vi "Remove All Aliases.vi"(8 "error in (no error)":errorcluster, 11 "Aliases Ref in":T1 format="%.0x") -> (0 "error out":errorcluster, 1 "Removed":bool, 3 "Aliases Ref out":T1 format="%.0x")   [LabVIEW 2017, in "Switch Scripting.lvlib"]
uses:
  Switch Scripting.lvlib
  <vilib>/NI Veristand/Custom Device API/Custom Device Item Ref.ctl
  <vilib>/NI VeriStand/Custom Device API/Custom Device API.lvlib
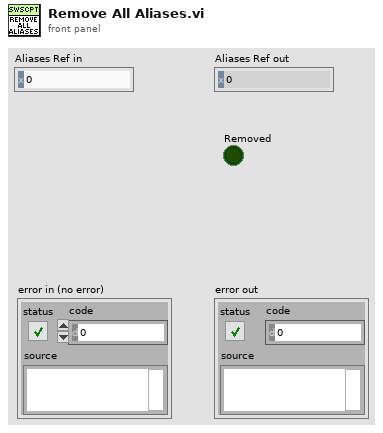
[diagram p1: front panel]
types:
  T1 = typedef "Custom Device API.lvlib/Custom Device Item Ref.ctl" = u64
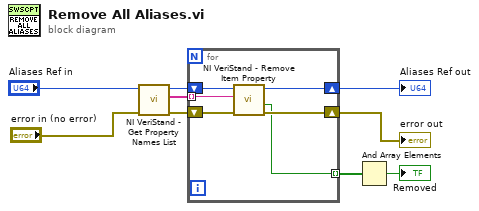
[diagram p0: block diagram]
diagram:
  n1 = call <vilib>:"NI VeriStand - Get Property Names List.vi"("error in (no error)"="error in (no error)", "Item Ref in"="Aliases Ref in") -> ("error out"=w8:errorcluster, "Property Names"=w9:string[], "Item Ref out"=w4:T1)  [unwired: 7 in]
  n2 = for {
    tunnel: w9 -> [w12] mode=indexing
    shift-right: [w13] -> w6
    shift-left: w8 -> [w15]
    shift-right: [w11] -> w3
    shift-left: w4 -> [w14]
    tunnel: [w10] -> w1 mode=indexing
    n3 = call <vilib>:"NI VeriStand - Remove Item Property.vi"("error in (no error)"=w15, "Property Name"=w12, "Item Ref in"=w14) -> ("error out"=w13:errorcluster, "Removed"=w10:bool, "Item Ref out"=w11:T1)  [unwired: 6 in]
  }
  "error out" <- w6
  "Aliases Ref out" <- w3
  n4 = And Array Elements(Boolean array=w1) -> (logical AND=→"Removed":bool)
